vi "RSZVB Automatic Vector Mixer Calibration.vi"(5 "Delay/Phase (0.0)":dbl format="%^.3e", 6 "Mixer Parameter (Auto)":i32(ring) items=["Auto", "User"], 7 "Dispersion (Off)":bool, 8 "error in (no error)":errorcluster {"code" format="%.0x"}, 9 "Mode (One-Port Calibration)":i32(ring) items=["One-Port Calibration", "Mixer Calibration"], 10 "Channel (1)":i32=1, 11 "VISA resource name":refnum<visa-resource-name>) -> (0 "error out":errorcluster {"code" format="%.0x"}, 3 "VISA resource name out":refnum<visa-resource-name>)   [LabVIEW 2011]
doc: "This VI allows the automatic vector mixer calibration using a calibration unit. It is only available in Vector Mixer Mode.\n\nNote(s):\n\n(1) The first part of the calibration (acquisition of one-port correction data using the calibration unit) is performed using :SENSE<Ch>:CORRECTION:COLLECT:AUTO:VMIXer:ACQuire BASE. Like in manual operation, the assignment between analyzer and calibration unit ports must be 1:1, i.e. analyzer ports 1 and 2 must be connected to calibration unit ports 1 and 2, respectively.\n\n(2) After connecting the reciprocal calibration mixer, the second part (acquisition of 2-port correction data) is performed using :SENSE<Ch>:CORRECTION:COLLECT:AUTO:VMIXer:ACQuire MIXer [, <Dispersion>, AUTO | <delay | phase>]. \n\n(3) Finally, to apply the resulting error terms to the related channel, use the RSZVB Calibration Auto Assignment Save.vi\n\nRemote-control command(s):\n[SENSe<Ch>:]CORRection:COLLect:AUTO:VMIXer:ACQuire BASE | MIXer [, <Dispersion>, AUTO | <delay | phase>]"
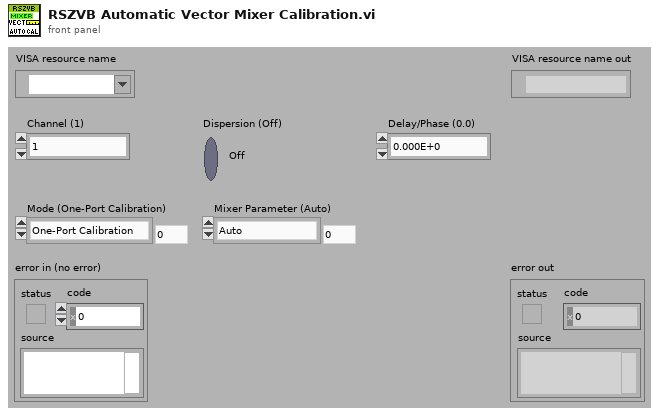
[diagram p1: front panel]
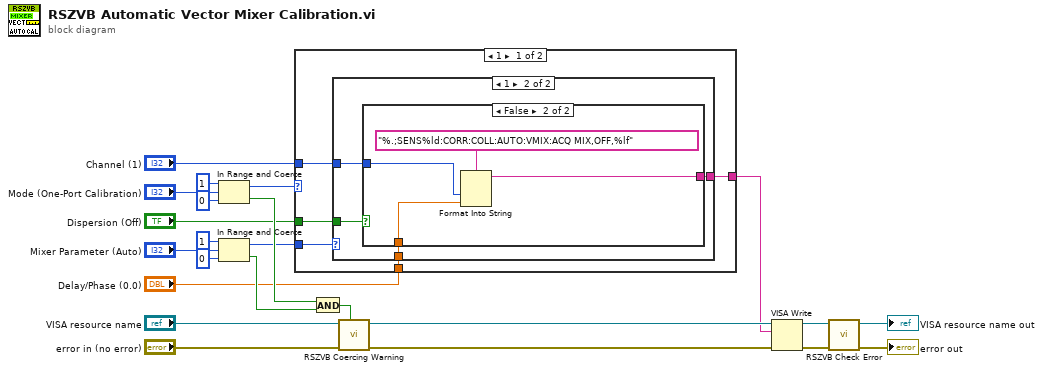
[diagram p0: block diagram]
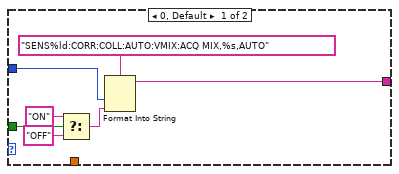
[diagram p2: hidden frame]
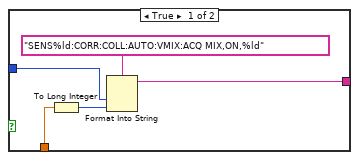
[diagram p3: hidden frame]
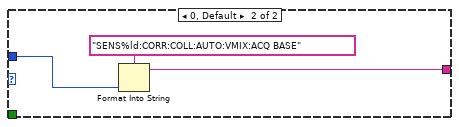
[diagram p4: hidden frame]
diagram:
  n1 = In Range and Coerce(upper limit=1, x="Mode (One-Port Calibration)", lower limit=0) -> (coerced(x)=w11:i32, In Range?=w9:bool)
  n2 = In Range and Coerce(upper limit=1, x="Mixer Parameter (Auto)", lower limit=0) -> (coerced(x)=w3:i32, In Range?=w5:bool)
  n3 = case shown="1" w11 {
    tunnel: [w28 w50] -> w17
    tunnel: "Channel (1)" -> [w26 w49]
    tunnel: w3 -> [w27 _]
    tunnel: "Dispersion (Off)" -> [w25 _]
    tunnel: "Delay/Phase (0.0)" -> [w24 _]
    frame 1 {
      n4 = case shown="1" w27 {
        tunnel: [w34 w39] -> w28
        tunnel: w26 -> [w33 w38]
        tunnel: w25 -> [w32 w37]
        tunnel: w24 -> [_ w36]
        frame 0, Default {
          n5 = Select(t="ON", s=w32, f="OFF") -> (s? t:f=w30:string)
          n6 = Format Into String(format string="SENS%ld:CORR:COLL:AUTO:VMIX:ACQ MIX,%s,AUTO", w33, w30) -> (resulting string=w34:string)  [unwired: 2 in, 1 out]
        }
        frame 1 {
          n7 = case shown="False" w37 {
            tunnel: [w43 w47] -> w39
            tunnel: w38 -> [w42 w46]
            tunnel: w36 -> [w41 w45]
            frame True {
              n8 = To Long Integer(number=w41) -> (32bit integer=w40:i32)
              n9 = Format Into String(format string="SENS%ld:CORR:COLL:AUTO:VMIX:ACQ MIX,ON,%ld", w42, w40) -> (resulting string=w43:string)  [unwired: 2 in, 1 out]
            }
            frame False {
              n10 = Format Into String(format string="%.;SENS%ld:CORR:COLL:AUTO:VMIX:ACQ MIX,OFF,%lf", w46, w45) -> (resulting string=w47:string)  [unwired: 2 in, 1 out]
            }
          }
        }
      }
    }
    frame 0, Default {
      n11 = Format Into String(format string="SENS%ld:CORR:COLL:AUTO:VMIX:ACQ BASE", w49) -> (resulting string=w50:string)  [unwired: 2 in, 1 out]
    }
  }
  n12 = And(x=w9, y=w5) -> (x .and. y?=w18:bool)
  n13 = call "RSZVB Coercing Warning.vi"("In Range?"=w18, "error in (no error)"="error in (no error)", "VISA session"="VISA resource name") -> ("error out"=w21:errorcluster, "dup VISA session"=w20:refnum<visa-resource-name>)  [unwired: 7 in]
  n14 = VISA Write(VISA resource name=w20, write buffer=w17, error in (no error)=w21) -> (VISA resource name out=w23:refnum<visa-resource-name>, error out=w22:errorcluster)  [unwired: 1 out]
  n15 = call "RSZVB Check Error.vi"("error in (no error)"=w22, "VISA session"=w23) -> ("error out"=→"error out":errorcluster, "dup VISA session"=→"VISA resource name out":refnum<visa-resource-name>)  [unwired: 8 in]
